vi "IIC Read Bytes Of Event.vi"(1 "TimeOutOfEventMs":i32, 4 "EventType":u8, 5 "EventPin":i32, 6 "ReadLen":i32, 7 "pReadData":u8[](array[numeric])=array[4097 elements], 9 "SlaveAddr":i16, 10 "IICIndex":i32, 11 "DevHandle":i32) -> (2 "function return":i32, 3 "pReadData out":u8[](array[numeric]))   [LabVIEW 2010, in "usb2iic.lvlib"]
doc: "int WINAPI IIC_ReadBytesOfEvent(int DevHandle,int IICIndex,short SlaveAddr,unsigned char *pReadData,int ReadLen,int EventPin,unsigned char EventType,int TimeOutOfEventMs);"
uses:
  usb2iic.lvlib
  USB2XXX.dll
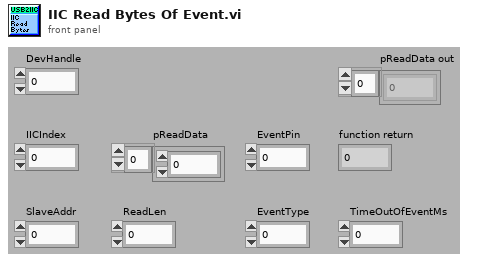
[diagram p1: front panel]
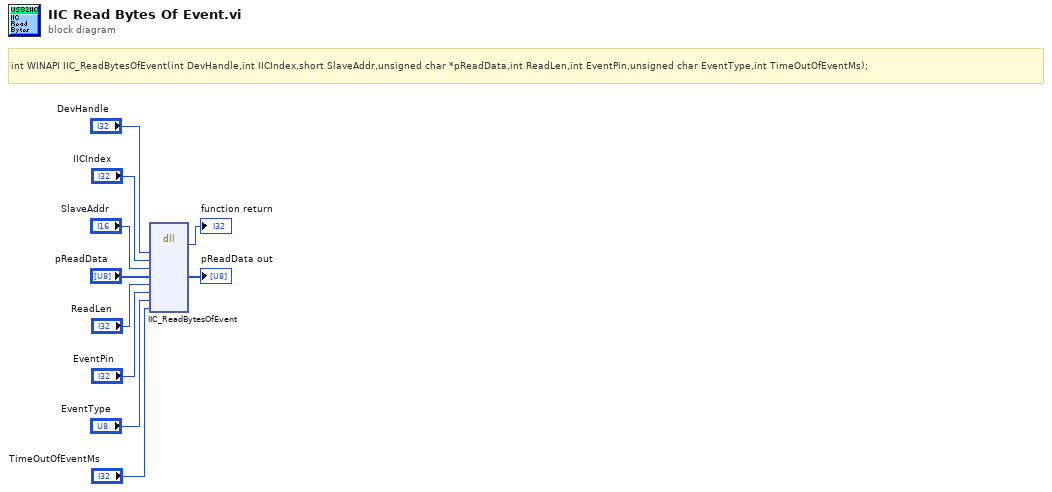
[diagram p0: block diagram]
diagram:
  # "int WINAPI IIC_ReadBytesOfEvent(int DevHandle,int IICIndex,short SlaveAddr,unsigned char *pReadData,int ReadLen,int EventPin,unsigned char EventType,int TimeOutOfEventMs);"
  n1 = dll-call lib="G:/OtherWork/USB2XXX_Example/trunk/Labview/PublicFiles/USB2XXX.*" fn="IIC_ReadBytesOfEvent"("DevHandle"="DevHandle", "IICIndex"="IICIndex", "SlaveAddr"="SlaveAddr", "pReadData"="pReadData", "ReadLen"="ReadLen", "EventPin"="EventPin", "EventType"="EventType", "TimeOutOfEventMs"="TimeOutOfEventMs") -> (→"function return":i32, "pReadData"=→"pReadData out":u8[])  [unwired: 10 in, 2 out]
